vi "OCV Initialize Camera.vi"(8 "error in (no error)":errorcluster, 11 "cam":i32) -> (0 "error out":errorcluster)   [LabVIEW 2018, in "OpenCVcamLV.lvlib"]
uses:
  OpenCVcamLV.lvlib
  LVopenCVcamDLL.dll
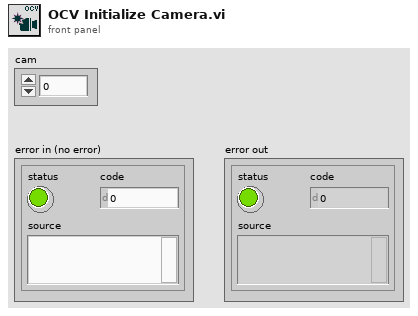
[diagram p1: front panel]
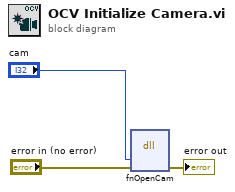
[diagram p0: block diagram]
diagram:
  n1 = dll-call lib="C:/Users/Andrey/Desktop/OpenCVcamLV/LVopenCVcamDLL.dll" fn="fnOpenCam"("cam"="cam", "err"="error in (no error)") -> ("err"=→"error out":errorcluster)  [unwired: 5 in, 2 out]
